vi "Actor Core.vi"(8 "error in":errorcluster, 11 "Example Actor in":refnum<class "Example Actor.lvclass">) -> (0 "error out":errorcluster, 3 "Actor out":refnum<class "Actor.lvclass">)   [LabVIEW 2016, in "Example Actor.lvclass"]
doc: "(<B>Filename</B>: Actor Framework.lvlib:Actor.lvclass:Actor Core.vi)\n\nReceives messages to the actor, reacts to them, and initiates any error handling that may shut the actor down.\n\nDescendant classes may override this VI to append parallel tasks for the actor to complete while it handles messages. Overrides use the Call Parent Method node.\n\n--\nCopyright © 2017 Composed SystemsI All rights reserved.\n\nAuthor: Jon McBee <jon.mcbee@composed.io>\n\nThis library is provided \"AS IS\" ,WITHOUT WARRANTIES OR\nCONDITIONS OF ANY KIND, either express or implied.\n\nComposed Systems -- composed.io\n\nStream 0.0.1.1\nJon McBee - Composed Systems\nCopyright (c) 2017, Composed Systems"
uses:
  <userlib>/Composed Systems/Stream/Mediator/Example/Example Actor/Example Actor.lvclass
  C:/Program Files (x86)/National Instruments/LabVIEW 2016/vi.lib/ActorFramework/Actor/Actor.lvclass
  <vilib>/ActorFramework/Actor/Actor.lvclass
  <userlib>/Composed Systems/Stream/Mediator/Example/Example Actor/Example Actor.lvclass/Example Actor.ctl
  <vilib>/ActorFramework/Actor/Actor.lvclass/Actor.ctl
  <vilib>/ActorFramework/Message Enqueuer/Message Enqueuer.lvclass/Message Enqueuer.ctl
  <vilib>/ActorFramework/Message Enqueuer/Init from Existing Queue.vi
  <vilib>/ActorFramework/Message Enqueuer/Enqueue.vi
  <vilib>/ActorFramework/Stop Msg/Stop Msg.lvclass
  C:/Program Files (x86)/National Instruments/LabVIEW 2016/vi.lib/ActorFramework/Message/Message.lvclass
  <vilib>/ActorFramework/Message Priority Queue/Priority Enqueue.vi
  <vilib>/ActorFramework/Message Enqueuer/Message Enqueuer.lvclass
panel:
  out "Data":dbl
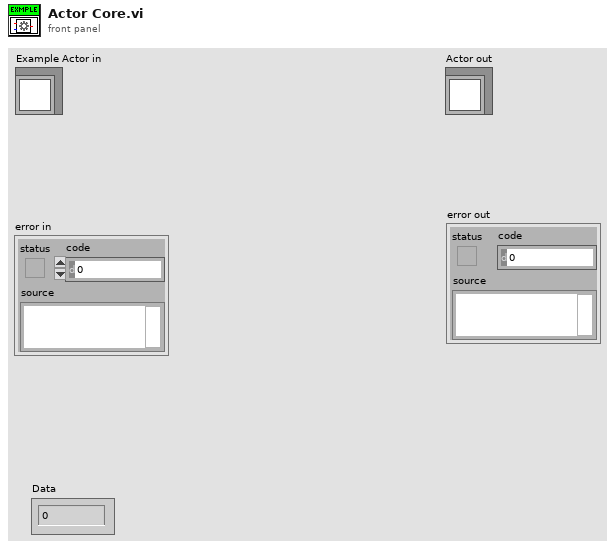
[diagram p1: front panel]
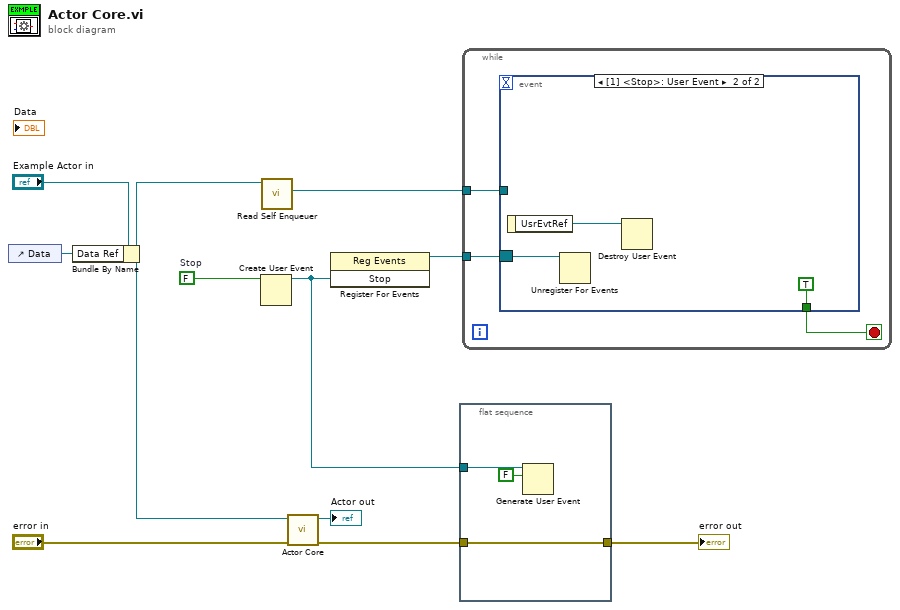
[diagram p0: block diagram]
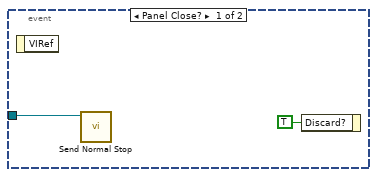
[diagram p2: hidden frame]
diagram:
  w9 = FALSE  # Stop
  n1 = control-ref of="Data"() -> (w1:refnum<vi>)
  n2 = Bundle By Name(cluster="Example Actor in", "Data Ref"=w1) -> (w2:refnum<class "Example Actor.lvclass">)
  n3 = Create User Event(user event datatype=w9) -> (user event=w5:refnum<user-event>)  [unwired: 1 in, 1 out]
  n4 = call <vilib>:"Read Self Enqueuer.vi"("Actor"=w2) -> ("Self Enqueuer"=w4:refnum<class "Message Enqueuer.lvclass">)  [unwired: 10 in]
  n5 = call-parent "Actor Core.vi"("error in"="error in", "Actor in"=w2) -> ("error out"=w7:errorcluster, "Actor out"=→"Actor out":refnum<class "Actor.lvclass">)  [unwired: 8 in]
  n6 = register-events(w5) -> (reference out=w8:refnum<event-registration>)  [unwired: 2 in, 1 out]
  n7 = flat-sequence {
    tunnel: w7 -> [w14]
    tunnel: [w14] -> w6
    tunnel: w5 -> [w13]
    frame #0 {
      n8 = Generate User Event(user event=w13, event data cluster=FALSE ("event data")) -> ()  [unwired: 2 in, 2 out]
    }
  }
  n9 = while {
    tunnel: w8 -> [w17]
    tunnel: w4 -> [w16]
    stop <- w15 stop-if-true
    n10 = event shown="[1] <Stop>: User Event" {
      selector: w17 -> [_ w21]
      dyn-events: _ -> [_ _]
      timeout: _ -> [_ _]
      tunnel: w16 -> [w18 _]
      tunnel: [_ TRUE] -> w15
      event Panel Close? {
        n11 = event-data() -> ()  [unwired: 1 in, 1 out]
        n12 = call <vilib>:"Send Normal Stop.vi"("Message Enqueuer"=w18) -> ()  [unwired: 10 in, 1 out]
        n13 = event-data("Discard?"=TRUE) -> ()  [unwired: 1 in, 1 out]
      }
      event User Event {
        n14 = event-data() -> ("UsrEvtRef"=w20:refnum<user-event>)  [unwired: 1 in]
        n15 = Unregister For Events(event registration refnum=w21) -> ()  [unwired: 1 in, 1 out]
        n16 = Destroy User Event(user event=w20) -> ()  [unwired: 1 in, 1 out]
      }
    }
  }
  "error out" <- w6
